vi "señal_seno_graph.vi"() -> ()   [LabVIEW 2020]
panel:
  in  "stop":bool
  out "Waveform Chart":dbl(graph)
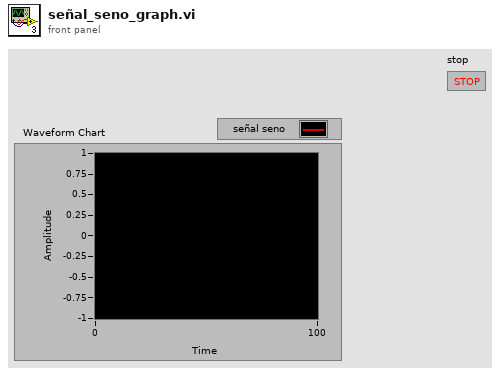
[diagram p1: front panel]
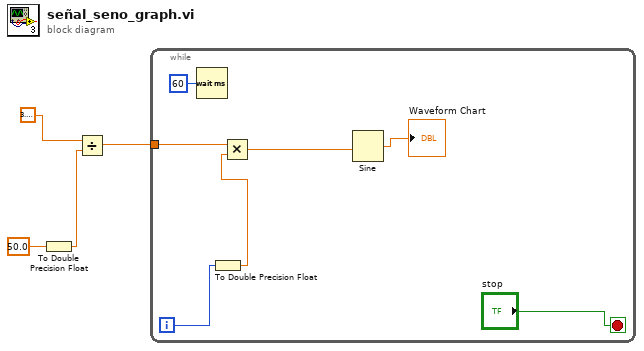
[diagram p0: block diagram]
diagram:
  n1 = To Double Precision Float(number=50.0) -> (double precision float=w2:dbl)
  n2 = Divide(x=3.141592653589793, y=w2) -> (x/y=w4:dbl)
  n3 = while {
    tunnel: w4 -> [w5]
    i -> [w6]
    stop <- "stop" stop-if-true
    n4 = Wait (ms)(milliseconds to wait=u32 60) -> ()  [unwired: 1 out]
    n5 = To Double Precision Float(number=w6) -> (double precision float=w7:dbl)
    n6 = Multiply(x=w5, y=w7) -> (x*y=w9:dbl)
    n7 = Sine(x=w9) -> (sin(x)=→"Waveform Chart":dbl)
  }
